vi "Item.vi"(8 "error in (no error)":errorcluster, 10 "Index":i32, 11 "BufferedArray in":refnum<class "BufferedArray.lvclass">) -> (0 "error out":errorcluster, 1 "Item":refnum<class>, 3 "BufferedArray out":refnum<class "BufferedArray.lvclass">)   [LabVIEW 2017, in "LapDog.Collections.v0.Lists.Implementations.lvlib" / "BufferedArray.lvclass"]
doc: "Returns a copy of the array element located at the given Index. If Index < 0 or Index > Cursor, a LVObject is returned."
uses:
  BufferedArray.lvclass
  BufferedArray.lvclass/BufferedArray.ctl
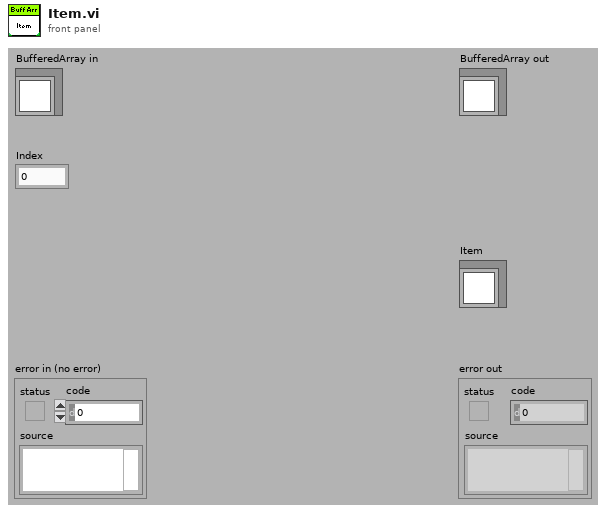
[diagram p1: front panel]
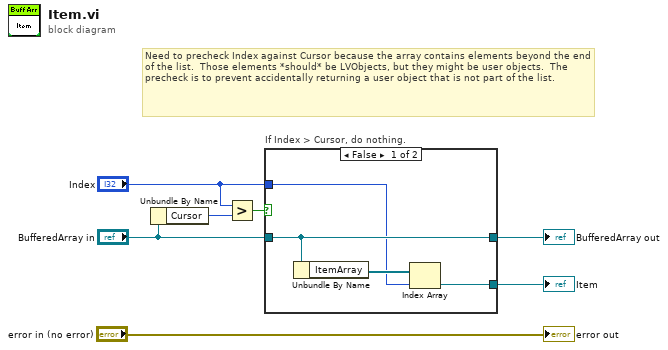
[diagram p0: block diagram]
diagram:
  # "Need to precheck Index against Cursor because the array contains elements beyond the end of the list.  Those elements *should* be LVObjects, but they might be user objects.  The precheck is to prevent accidentally returning a user object that is not part of the list."
  n1 = Unbundle By Name("BufferedArray in") -> ("Cursor"=w6:i32)
  n2 = Greater?(x="Index", y=w6) -> (0:w5:bool)
  n3 = case "If Index > Cursor, do nothing." shown="False" w5 {
    tunnel: "BufferedArray in" -> [w11 w12]
    tunnel: [w11 w12] -> w3
    tunnel: "Index" -> [w9 _]
    tunnel: [w8 _] -> w1
    frame False {
      n4 = Unbundle By Name(w11) -> ("ItemArray"=w10:refnum<class>[])
      n5 = Index Array(array=w10, index=w9) -> (element=w8:refnum<class>)
    }
    frame True {
    }
  }
  "BufferedArray out" <- w3
  "Item" <- w1
  "error out" <- "error in (no error)"
